vi "node3.vi"(11 "State in":T1) -> ()   [LabVIEW 2012]
uses:
  <vilib>/Embedded/WSN/WSNState.ctl
  <vilib>/Embedded/WSN/OperatingMode.ctl
  <vilib>/Embedded/WSN/EIO/NI WSN-3202/EIO Prop Node Gain.ctl
  <vilib>/Embedded/WSN/EIO/NI WSN-3202/WSN-3202 EIO Prop Node DIO Drive Mode.ctl
  <vilib>/Embedded/WSN/Error codes.ctl
  <vilib>/LabVIEW Targets/Embedded/WSN/Config Node.xnode
  <vilib>/eio/EIOPropertyNode/EIOPropertyNode.xnode
  <vilib>/eio/EIONode/EIONode.xnode
  <vilib>/LabVIEW Targets/Embedded/WSN/RadioMessages.xnode
types:
  T1 = typedef "WSNState.ctl" = enum16{"Start", "Sample", "Receive", "Network Status Change", "DIO Notification"}
  T2 = typedef "OperatingMode.ctl" = enum32{"Host Driven", "VI Driven"}
  T3 = typedef "WSN-3202 EIO Prop Node DIO Drive Mode.ctl" = u16
  T4 = typedef "EIO Prop Node Gain.ctl" = u16
  T5 = cluster{"mod":i32, "bat":i32, "pow":i32, "sh1":i32, "sh2":i32}
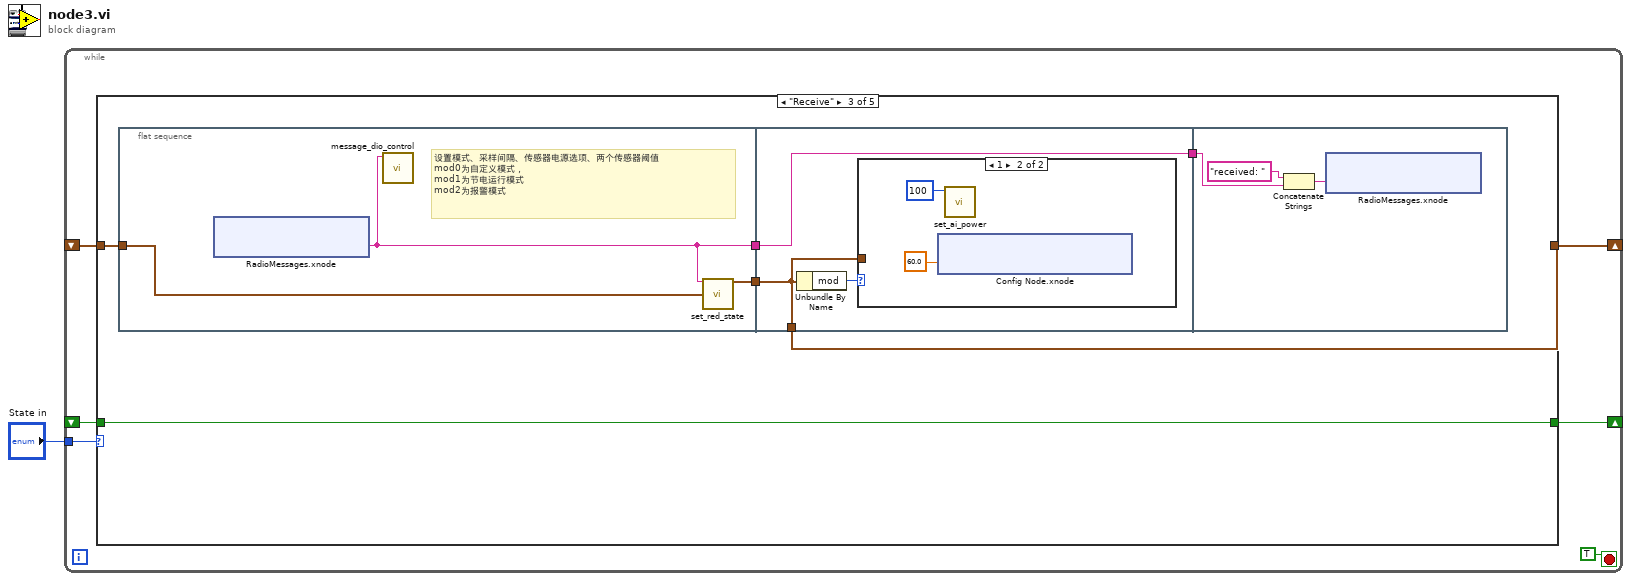
[diagram p0: block diagram]
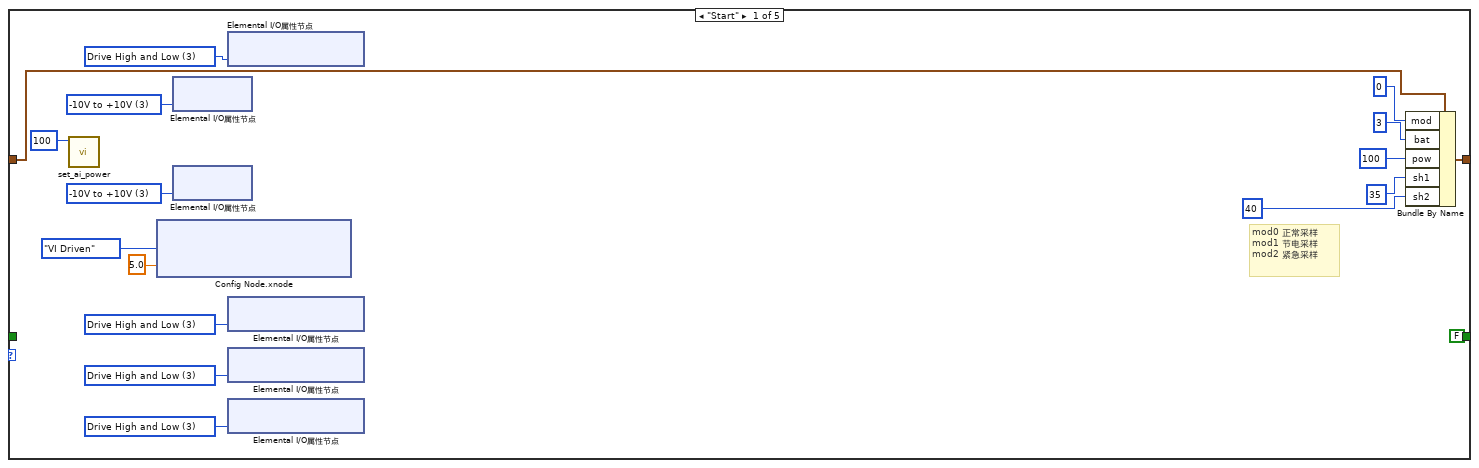
[diagram p2: hidden frame]
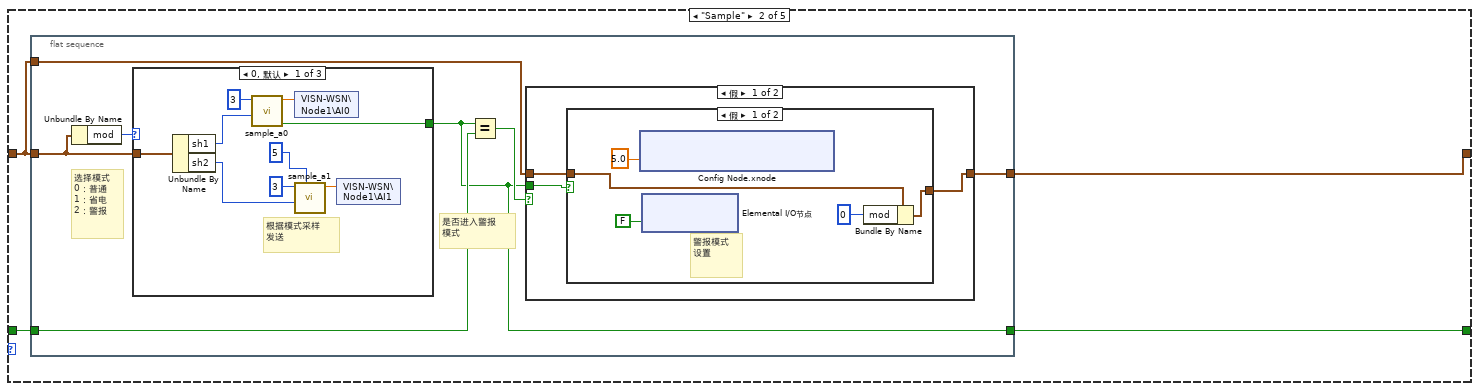
[diagram p3: hidden frame]
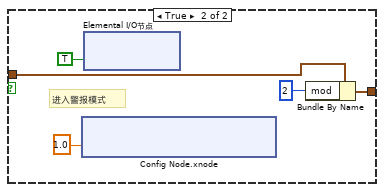
[diagram p4: hidden frame]
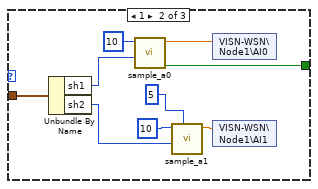
[diagram p6: hidden frame]
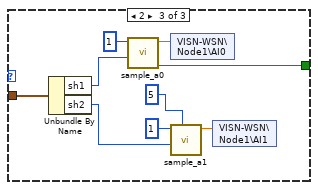
[diagram p7: hidden frame]
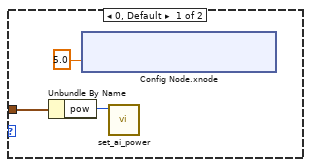
[diagram p8: hidden frame]
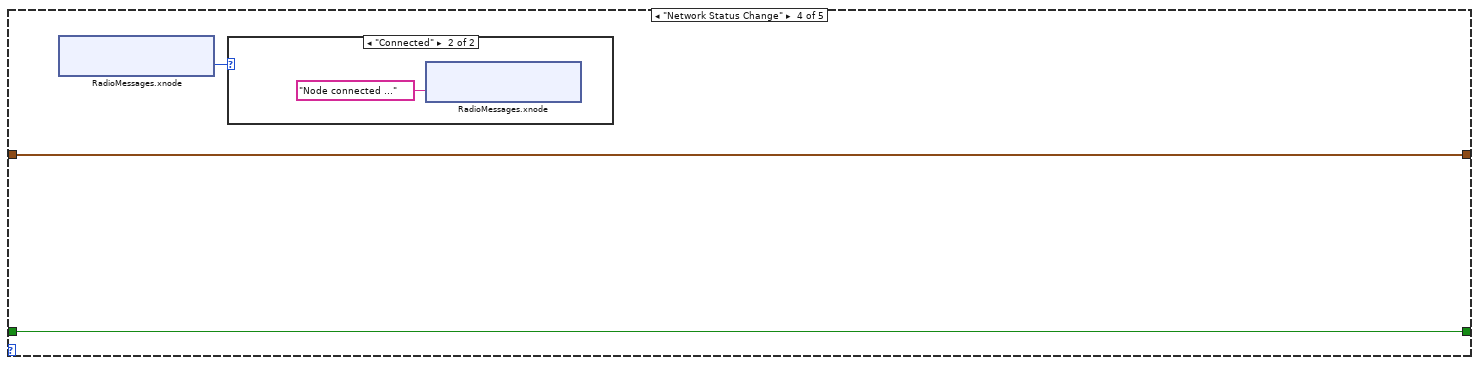
[diagram p9: hidden frame]
diagram:
  n1 = while {
    tunnel: "State in" -> [w7]
    shift-right: [w5] -> _
    shift-left: _ -> [w4]
    shift-right: [w2] -> _
    shift-left: _ -> [w3]
    stop <- TRUE stop-if-true
    n2 = case shown="\"Receive\"" w7 {
      tunnel: [w9 w43 w116 w157 w170] -> w5
      tunnel: w4 -> [w10 w44 w117 w157 w170]
      tunnel: w3 -> [_ w41 w115 w156 w169]
      tunnel: [FALSE ("布尔") w42 w115 w156 w169] -> w2
      frame "Start" {
        w17 = T3 3 items=["Host Driven"=65535, "Tristate"=0, "Drive Low Only"=1, "Drive High Only"=2, "Drive High and Low"=3] ("DIO Drive Mode")
        w18 = T3 3 items=["Host Driven"=65535, "Tristate"=0, "Drive Low Only"=1, "Drive High Only"=2, "Drive High and Low"=3] ("DIO Drive Mode")
        w19 = T3 3 items=["Host Driven"=65535, "Tristate"=0, "Drive Low Only"=1, "Drive High Only"=2, "Drive High and Low"=3] ("DIO Drive Mode")
        w20 = T3 3 items=["Host Driven"=65535, "Tristate"=0, "Drive Low Only"=1, "Drive High Only"=2, "Drive High and Low"=3] ("DIO Drive Mode")
        w21 = T4 3 items=["Host Driven"=65535, "-10V to +10V"=3, "-5V to +5V"=5, "-2V to +2V"=130, "-0.5V to +0.5V"=131] ("Range")
        w22 = T4 3 items=["Host Driven"=65535, "-10V to +10V"=3, "-5V to +5V"=5, "-2V to +2V"=130, "-0.5V to +0.5V"=131] ("Range")
        # "mod0 正常采样\nmod1 节电采样\nmod2 紧急采样"
        n3 = call "set_ai_power.vi"("pow"=100) -> ()  [unwired: 11 in]
        n4 = xnode "Config Node.xnode"("sampleIntervalMode"=OperatingMode."VI Driven" ("sampleRateMode"), "sampleInterval"=sgl 5.0 ("sampleRate")) -> ()  [unwired: 1 in, 1 out]
        n5 = xnode "Elemental I/O属性节点"("Range"=w21) -> ()  [unwired: 1 in, 1 out]
        n6 = xnode "Elemental I/O属性节点"("Range"=w22) -> ()  [unwired: 1 in, 1 out]
        n7 = xnode "Elemental I/O属性节点"("DIO Drive Mode"=w18) -> ()  [unwired: 1 in, 1 out]
        n8 = xnode "Elemental I/O属性节点"("DIO Drive Mode"=w17) -> ()  [unwired: 1 in, 1 out]
        n9 = xnode "Elemental I/O属性节点"("DIO Drive Mode"=w19) -> ()  [unwired: 1 in, 1 out]
        n10 = xnode "Elemental I/O属性节点"("DIO Drive Mode"=w20) -> ()  [unwired: 1 in, 1 out]
        n11 = Bundle By Name(cluster=w10, "mod"=0, "bat"=3, "pow"=100, "sh1"=35, "sh2"=40) -> (w9:T5)
      }
      frame "Sample" {
        n12 = flat-sequence {
          tunnel: [w48] -> w43
          tunnel: w44 -> [w49]
          tunnel: w44 -> [w50]
          tunnel: [w45] -> w42
          tunnel: w41 -> [w47]
          frame #0 {
            # "是否进入警报\n模式"
            # "选择模式\n0：普通\n1：省电\n2：警报"
            n13 = Unbundle By Name(w50) -> ("mod"=w51:i32)
            n14 = case shown="0, 默认" w51 {
              tunnel: [w89 w98 w107] -> w45
              tunnel: w50 -> [w92 w101 w106]
              frame 0, Default {
                # "根据模式采样\n发送"
                n15 = Unbundle By Name(w92) -> ("sh1"=w91:i32, "sh2"=w90:i32)
                n16 = call "sample_a0.vi"("threshold"=w91, "times"=3) -> ("布尔"=w89:bool, "ai"=w93:sgl)  [unwired: 8 in]
                n17 = shared-variable "VISN-WSN\\Node1\\AI0"(w93) -> ()  [unwired: 1 in, 1 out]
                n18 = call "sample_a1.vi"("delta"=5, "threshold"=w90, "times"=3) -> ("ai"=w94:sgl)  [unwired: 8 in]
                n19 = shared-variable "VISN-WSN\\Node1\\AI1"(w94) -> ()  [unwired: 1 in, 1 out]
              }
              frame 1 {
                n20 = Unbundle By Name(w101) -> ("sh1"=w100:i32, "sh2"=w99:i32)
                n21 = call "sample_a0.vi"("threshold"=w100, "times"=10) -> ("布尔"=w98:bool, "ai"=w103:sgl)  [unwired: 8 in]
                n22 = call "sample_a1.vi"("delta"=5, "threshold"=w99, "times"=10) -> ("ai"=w102:sgl)  [unwired: 8 in]
                n23 = shared-variable "VISN-WSN\\Node1\\AI0"(w103) -> ()  [unwired: 1 in, 1 out]
                n24 = shared-variable "VISN-WSN\\Node1\\AI1"(w102) -> ()  [unwired: 1 in, 1 out]
              }
              frame 2 {
                n25 = Unbundle By Name(w106) -> ("sh1"=w112:i32, "sh2"=w113:i32)
                n26 = call "sample_a0.vi"("threshold"=w112, "times"=1) -> ("布尔"=w107:bool, "ai"=w110:sgl)  [unwired: 8 in]
                n27 = shared-variable "VISN-WSN\\Node1\\AI0"(w110) -> ()  [unwired: 1 in, 1 out]
                n28 = call "sample_a1.vi"("delta"=5, "threshold"=w113, "times"=1) -> ("ai"=w111:sgl)  [unwired: 8 in]
                n29 = shared-variable "VISN-WSN\\Node1\\AI1"(w111) -> ()  [unwired: 1 in, 1 out]
              }
            }
            n30 = Equal?(x=w45, y=w47) -> (x = y?=w46:bool)
            n31 = case shown="假" w46 {
              tunnel: w49 -> [w54 w87]
              tunnel: [w53 w87] -> w48
              tunnel: w45 -> [w52 _]
              frame False {
                n32 = case shown="假" w52 {
                  tunnel: w54 -> [w58 w75]
                  tunnel: [w57 w73] -> w53
                  frame False {
                    # "警报模式\n设置"
                    n33 = xnode "Config Node.xnode"("sampleInterval"=sgl 5.0) -> ()  [unwired: 1 in, 1 out]
                    n34 = xnode "Elemental I/O节点"("User LED"=FALSE ("bell")) -> ()  [unwired: 1 in, 1 out]
                    n35 = Bundle By Name(cluster=w58, "mod"=0) -> (w57:T5)
                  }
                  frame True {
                    # "进入警报模式"
                    n36 = xnode "Config Node.xnode"("sampleInterval"=sgl 1.0) -> ()  [unwired: 1 in, 1 out]
                    n37 = xnode "Elemental I/O节点"("User LED"=TRUE ("bell")) -> ()  [unwired: 1 in, 1 out]
                    n38 = Bundle By Name(cluster=w75, "mod"=2) -> (w73:T5)
                  }
                }
              }
              frame True {
              }
            }
          }
        }
      }
      frame "Receive" {
        n39 = flat-sequence {
          tunnel: [w123] -> w119
          tunnel: [w122] -> w118
          tunnel: w117 -> [w121]
          tunnel: [w136] -> w120
          tunnel: w119 -> [w136]
          tunnel: w118 -> [w134]
          tunnel: [w134] -> w116
          tunnel: w120 -> [w148]
          frame #0 {
            # "设置模式、采样间隔、传感器电源选项、两个传感器阈值\nmod0为自定义模式，\nmod1为节电运行模式\nmod2为报警模式"
            n40 = xnode "RadioMessages.xnode"() -> ("receivedUserMessage"=w123:string)  [unwired: 2 out]
            n41 = call "message_dio_control.vi"("usermessage"=w123) -> ()  [unwired: 11 in]
            n42 = call "set_red_state.vi"("字符串"=w123, "red"=w121) -> ("set"=w122:T5)  [unwired: 13 in]
          }
          frame #1 {
            n43 = Unbundle By Name(w134) -> ("mod"=w135:i32)
            n44 = case shown="1" w135 {
              tunnel: w134 -> [w138 _]
              frame 0, Default {
                n45 = Unbundle By Name(w138) -> ("pow"=w137:i32)
                n46 = xnode "Config Node.xnode"("sampleInterval"=sgl 5.0) -> ()  [unwired: 1 in, 1 out]
                n47 = call "set_ai_power.vi"("pow"=w137) -> ()  [unwired: 11 in]
              }
              frame 1 {
                n48 = xnode "Config Node.xnode"("sampleInterval"=sgl 60.0) -> ()  [unwired: 1 in, 1 out]
                n49 = call "set_ai_power.vi"("pow"=100) -> ()  [unwired: 11 in]
              }
            }
          }
          frame #2 {
            n50 = Concatenate Strings("received: ", w148) -> (w150:string)
            n51 = xnode "RadioMessages.xnode"("sendDebugMessage"=w150) -> ()  [unwired: 2 out]
          }
        }
      }
      frame "Network Status Change" {
        n52 = xnode "RadioMessages.xnode"() -> ("networkStatus"=w158:enum16{"Disconnected", "Connected"})  [unwired: 2 out]
        n53 = case shown="\"Connected\"" w158 {
          frame "Disconnected", Default {
          }
          frame "Connected" {
            n54 = xnode "RadioMessages.xnode"("sendDebugMessage"="Node connected ...") -> ()  [unwired: 2 out]
          }
        }
      }
      frame "DIO Notification" {
      }
    }
  }
